vi "refnum names.vi"() -> ()   [LabVIEW 2015]
panel:
  out "AdaFruit IMU Orient":string="Deploy Pins"
  out "Deploy Pins":string="Deploy Pins"
  out "Right Slave":string="Right Slave"
  out "Left Slave":string="Left Slave"
  out "Right LEDs":string="Right LEDs"
  out "Left LEDs":string="Left LEDs"
  out "Inner LEDs":string="Inner LEDs"
  out "Left Catapult Limit Switch":string="Left Catapult Limit Switch"
  out "Gamepad 1":string="Gamepad 1"
  out "Forward IR Sensor":string="Forward IR Sensor"
  out "Right IR Sensor":string="Right IR Sensor"
  out "Left IR Sensor":string="Left IR Sensor"
  out "Right Catapult Limit Switch":string="Right Catapult Limit Switch"
  out "Gyro":string="Gyro"
  out "Climb Arm Deploy Motor":string="Climb Arm Deploy Motor"
  out "Lift/Drive Shifter":string="Lift/Drive Shifter"
  out "Ball Lifter Left":string="Ball Lifter Left"
  out "Ball Grabber Motor":string="Ball Grabber Motor"
  out "Ball Lifter Right":string="Ball Lifter Right"
  out "Catapult Trigger":string="Catapult Trigger"
  out "Catapult Winch Motor":string="Catapult Winch Motor"
  out "Right Master":string="Right Master"
  out "Gamepad 0":string="Gamepad 0"
  out "Left Master":string="Left Master"
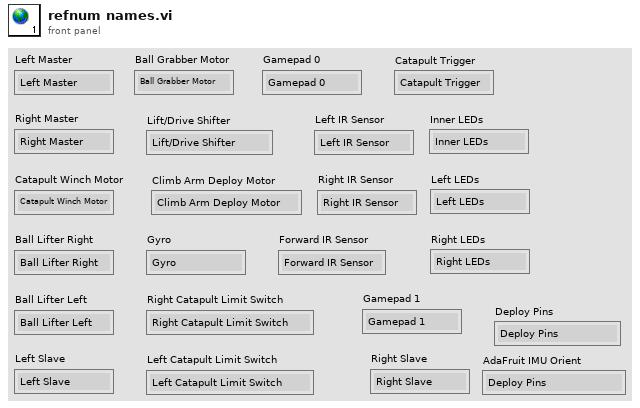
[diagram p1: front panel]
diagram:
